vi "Pause Processing.vi"(8 "error in (no error)":errorcluster, 10 "Internal Message Queue":refnum<queue>) -> (0 "error out":errorcluster)   [LabVIEW 2023, in "HAF.lvlib" / "InteractionProcessor.lvclass"]
doc: "Clear the Internal queue and wait for a Resume message to appear. The queue is reset as Pause messages are raised at the front of the queue (high priority) and no messages originally in the queue should be processed.\n\nProcessing only pauses after the current run through of Command Directors completes."
uses:
  InteractionProcessor.lvclass
  Message.ctl
  InteractionProcessor.lvclass/InteractionProcessor.ctl
  HAF.lvlib
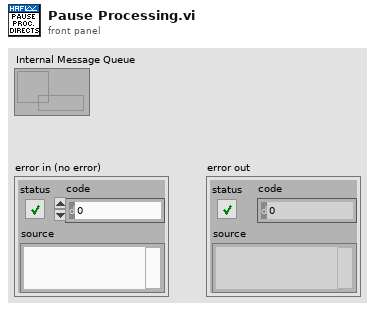
[diagram p1: front panel]
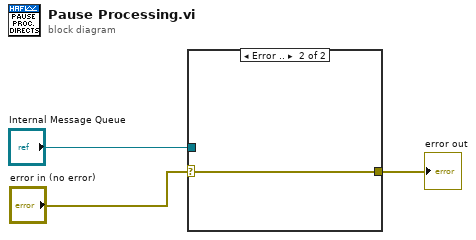
[diagram p0: block diagram]
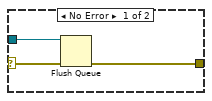
[diagram p2: hidden frame]
diagram:
  n1 = case shown="Error .." "error in (no error)" {
    selector: "error in (no error)" -> [w4 w7]
    tunnel: [w6 w7] -> w3
    tunnel: "Internal Message Queue" -> [w5 _]
    frame No Error {
      n2 = Flush Queue(queue=w5, error in (no error)=w4) -> (error out=w6:errorcluster)  [unwired: 2 out]
    }
    frame Error {
    }
  }
  "error out" <- w3
